vi "Project Tree Drop.vi"(8 "error in (no error)":errorcluster, 9 "Available Data Names":string[](array[string]), 10 "Coords":T2, 11 "TreeControl in":refnum<vi>) -> (0 "error out":errorcluster, 2 "Drop Event Data":T1, 3 "Valid":bool)   [LabVIEW 2015, in "Editor.lvclass"]
uses:
  Editor.lvclass
  <vilib>/Utility/miscctls.llb/LVPoint32TypeDef.ctl
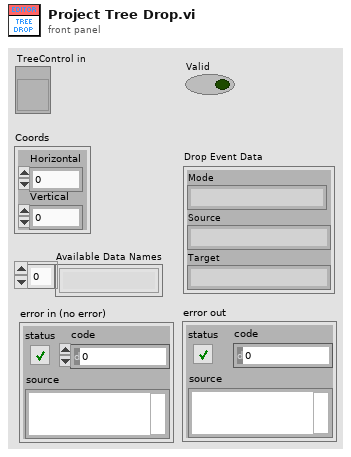
[diagram p1: front panel]
types:
  T1 = cluster{"Mode":string, "Source":string, "Target":string}
  T2 = typedef "LVPoint32TypeDef.ctl" = cluster{"Horizontal":i32, "Vertical":i32}
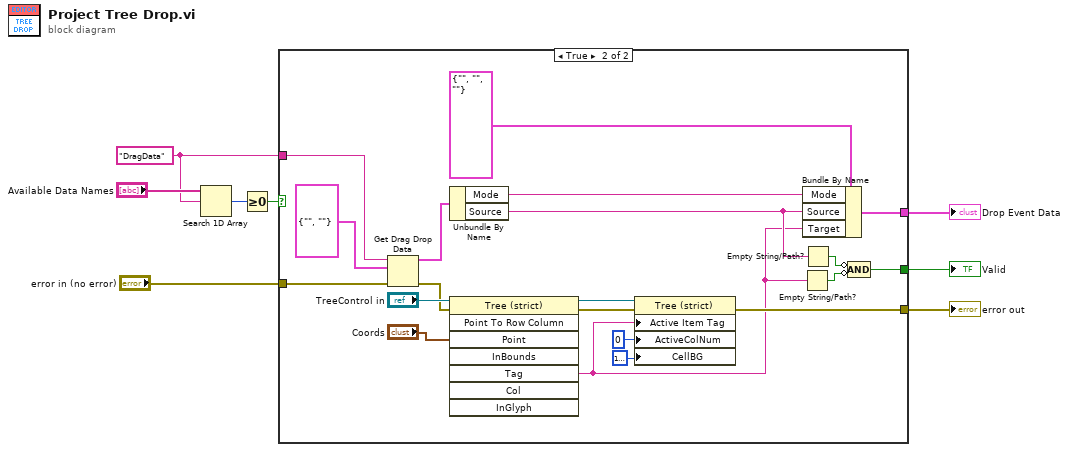
[diagram p0: block diagram]
diagram:
  w6 = "DragData" ("data name")
  n1 = Search 1D Array(1D array="Available Data Names", element=w6) -> (index of element=w5:i32)  [unwired: 1 in]
  n2 = Greater Or Equal To 0?(x=w5) -> (x >= 0?=w4:bool)
  n3 = case shown="True" w4 {
    tunnel: "error in (no error)" -> [w9 w26]
    tunnel: w6 -> [_ w24]
    tunnel: [w9 w11] -> w3
    tunnel: [_ w20] -> w2
    tunnel: [_ w16] -> w1
    frame False {
    }
    frame True {
      n4 = Get Drag Drop Data(6:w26, 8:cluster{"Mode":string, "Source":string} {"Mode"="", "Source"=""}, 9:w24) -> (0:w25:errorcluster, 3:w23:cluster{"Mode":string, "Source":string})
      n5 = Unbundle By Name(w23) -> ("Mode"=w18:string, "Source"=w17:string)
      n6 = invoke class="Tree (strict)" method="Point To Row Column"(reference="TreeControl in", error in=w25, "Point"="Coords") -> (reference out=w13:refnum<vi>, error out=w12:errorcluster, "Tag"=w10:string)  [unwired: 5 in, 5 out]
      n7 = property class="Tree (strict)"(reference=w13, error in=w12, "Active Item Tag"=w10, "ActiveColNum"=0 ("Active Cell:Active Column Number"), "CellBG"=u32 16777216) -> (error out=w11:errorcluster)  [unwired: 1 out]
      n8 = Empty String/Path?(string/path=w10) -> (empty?=w21:bool)
      n9 = Bundle By Name(cluster=T1 {"Mode"="", "Source"="", "Target"=""} ("Drop Event Data"), "Mode"=w18, "Source"=w17, "Target"=w10) -> (w16:T1)
      n10 = Empty String/Path?(string/path=w17) -> (empty?=w22:bool)
      n11 = Compound Arithmetic op=AND(invert w22, invert w21) -> (w20:bool)
    }
  }
  "Valid" <- w2
  "error out" <- w3
  "Drop Event Data" <- w1
